vi "PCC Activate.vi"(8 "error in (no error)":errorcluster, 10 "Frequency Control":refnum<class "Message Enqueuer.lvclass">, 11 "IED in":refnum<class "IED.lvclass">) -> (0 "error out":errorcluster, 3 "IED out":refnum<class "IED.lvclass">)   [LabVIEW 2015, in "IED Actor.lvlib" / "IED.lvclass"]
uses:
  IED.lvclass
  <vilib>/ActorFramework/Message Enqueuer/Message Enqueuer.lvclass
  IED.lvclass/IED.ctl
  SCADA Core/SCADA Abstract Messages/Simple Command Status Msg/Simple Command Status.ctl
  <vilib>/ActorFramework/Actor/Actor.lvclass/Actor.ctl
  SCADA Core/SCADA Response Messages/Return Activate Status Msg/Return Activate Status Msg.lvclass/Return Activate Status Msg.ctl
  <vilib>/ActorFramework/Message Enqueuer/Message Enqueuer.lvclass/Message Enqueuer.ctl
  <vilib>/ActorFramework/Message Enqueuer/Enqueue.vi
  <vilib>/ActorFramework/Message Priority Queue/Priority Enqueue.vi
  SCADA Core/SCADA Response Messages/Return Activate Status Msg/Return Activate Status Msg.lvclass
  SCADA Core/SCADA Messages/Grid Activate Msg/Grid Activate Msg.lvclass
  <vilib>/Modbus/master/Modbus Master.lvclass
  <vilib>/ActorFramework/Actor/Actor.lvclass
  SCADA Core/SCADA Abstract Messages/Simple Command Status Msg/Simple Command Status Msg.lvclass
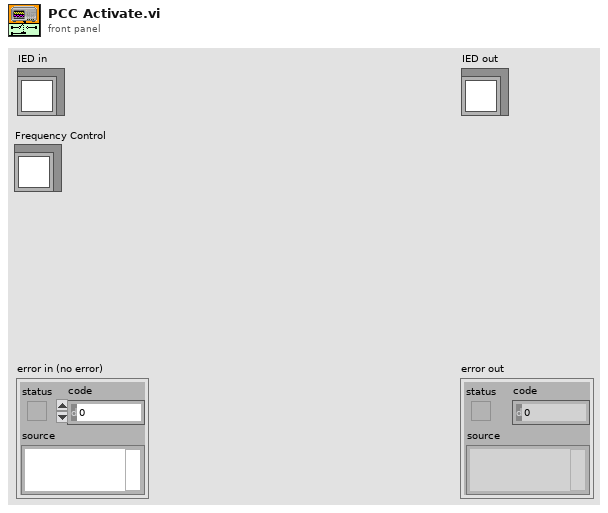
[diagram p1: front panel]
types:
  T1 = typedef "SCADA Core.lvlib/Simple Command Status Msg.lvclass/Simple Command Status.ctl" = enum16{"Success", "Failure"}
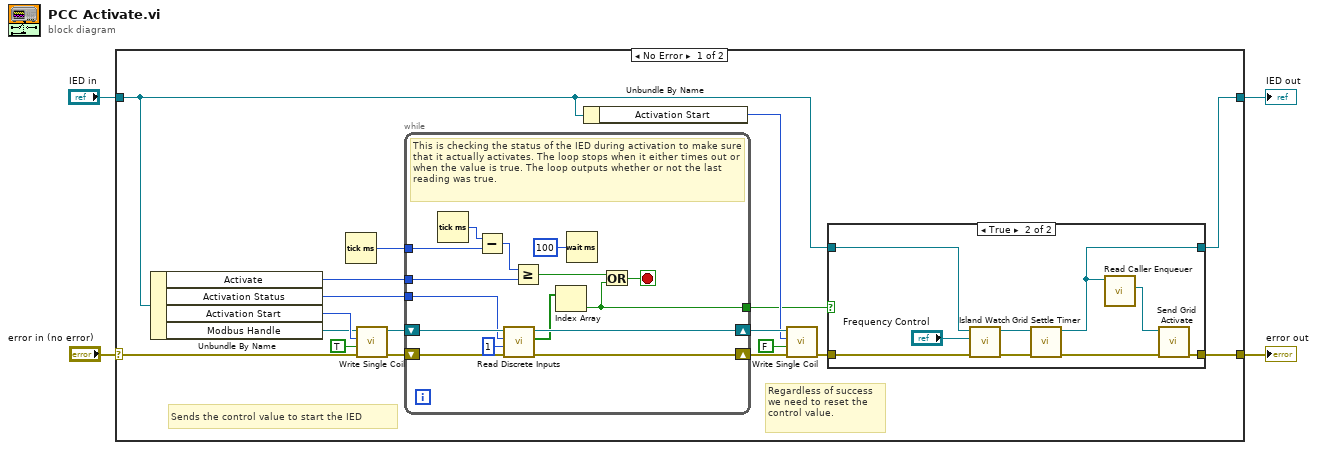
[diagram p0: block diagram]
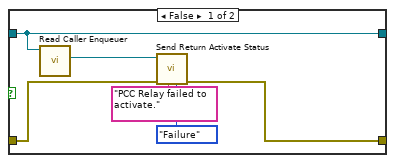
[diagram p2: hidden frame]
diagram:
  n1 = case shown="No Error" "error in (no error)" {
    selector: "error in (no error)" -> [w7 w54]
    tunnel: [w10 w54] -> w2
    tunnel: [w8 w53] -> w3
    tunnel: "IED in" -> [w9 w53]
    frame No Error {
      # "Regardless of success we need to reset the control value."
      # "Sends the control value to start the IED"
      n2 = Unbundle By Name(w9) -> ("Activate"=w16:u32, "Activation Status"=w17:u16, "Activation Start"=w21:u16, "Modbus Handle"=w6:refnum<class "Modbus Master.lvclass">)
      n3 = Tick Count (ms)() -> (millisecond timer value=w22:u32)
      n4 = call-dynamic "Write Single Coil.vi"("error in (no error)"=w7, "coil value"=TRUE, "address"=w21, "Modbus master in"=w6) -> ("error out"=w18:errorcluster, "Modbus master out"=w19:refnum<class "Modbus Master.lvclass">)  [unwired: 6 in]
      n5 = while {
        tunnel: w22 -> [w50]
        tunnel: w16 -> [w48]
        tunnel: w17 -> [w44]
        shift-right: [w38] -> w15
        shift-left: w18 -> [w43]
        tunnel: [w39] -> w11
        shift-right: [w41] -> w14
        shift-left: w19 -> [w45]
        stop <- w46 stop-if-true
        # "This is checking the status of the IED during activation to make sure that it actually activates. The loop stops when it either times out or when the value is true. The loop outputs whether or not the last reading was true."
        n6 = Tick Count (ms)() -> (millisecond timer value=w51:u32)
        n7 = Subtract(x=w51, y=w50) -> (x-y=w49:u32)
        n8 = call-dynamic "Read Discrete Inputs.vi"("error in (no error)"=w43, "number of discrete inputs"=u16 1 ("number of coils"), "starting address"=w44, "Modbus master in"=w45) -> ("error out"=w38:errorcluster, "discrete input values"=w40:bool[], "Modbus master out"=w41:refnum<class "Modbus Master.lvclass">)  [unwired: 5 in]
        n9 = Greater Or Equal?(x=w49, y=w48) -> (x >= y?=w47:bool)
        n10 = Index Array(array=w40) -> (element=w39:bool)  [unwired: 1 in]
        n11 = Wait (ms)(milliseconds to wait=u32 100) -> ()  [unwired: 1 out]
        n12 = Or(x=w47, y=w39) -> (x .or. y?=w46:bool)
      }
      n13 = Unbundle By Name(w9) -> ("Activation Start"=w13:u16)
      n14 = call-dynamic "Write Single Coil.vi"("error in (no error)"=w15, "coil value"=FALSE, "address"=w13, "Modbus master in"=w14) -> ("error out"=w5:errorcluster)  [unwired: 6 in, 1 out]
      n15 = case shown="True" w11 {
        tunnel: w5 -> [w27 w34]
        tunnel: w9 -> [w23 w35]
        tunnel: [w26 w37] -> w10
        tunnel: [w23 w31] -> w8
        frame False {
          n16 = call <vilib>:"Read Caller Enqueuer.vi"("Actor"=w23) -> ("Caller Enqueuer"=w28:refnum<class "Message Enqueuer.lvclass">)  [unwired: 10 in]
          n17 = call "Send Return Activate Status.vi"("Status"=Simple_Command_Status."Failure", "error"="PCC Relay failed to activate.", "error in (no error)"=w27, "Message Enqueuer"=w28) -> ("error out"=w26:errorcluster)  [unwired: 6 in, 1 out]
        }
        frame True {
          n18 = call "Island Watch.vi"("error in (no error)"=w34, "Frequency Control"="Frequency Control", "IED in"=w35) -> ("error out"=w30:errorcluster, "IED out"=w32:refnum<class "IED.lvclass">)  [unwired: 7 in]
          n19 = call "Grid Settle Timer.vi"("error in (no error)"=w30, "IED in"=w32) -> ("error out"=w29:errorcluster, "IED out"=w31:refnum<class "IED.lvclass">)  [unwired: 8 in]
          n20 = call <vilib>:"Read Caller Enqueuer.vi"("Actor"=w31) -> ("Caller Enqueuer"=w36:refnum<class "Message Enqueuer.lvclass">)  [unwired: 10 in]
          n21 = call "Send Grid Activate.vi"("error in (no error)"=w29, "Message Enqueuer"=w36) -> ("error out"=w37:errorcluster)  [unwired: 8 in, 1 out]
        }
      }
    }
    frame Error {
    }
  }
  "error out" <- w2
  "IED out" <- w3
